vi "Read Stage Model And Serial Number.vi"(4 "error in (no error)":errorcluster, 7 "VISA resource name":refnum<visa-resource-name>) -> (0 "error out":errorcluster, 1 "Serial number":string, 2 "Model number":string, 3 "VISA resource name out":refnum<visa-resource-name>)   [LabVIEW 2020, in "Newport ESP301.lvlib"]
doc: "Reads the stage model and the serial number."
uses:
  Newport ESP301.lvlib
panel:
  in  "Axis (1)":i32=1 min=1 max=3
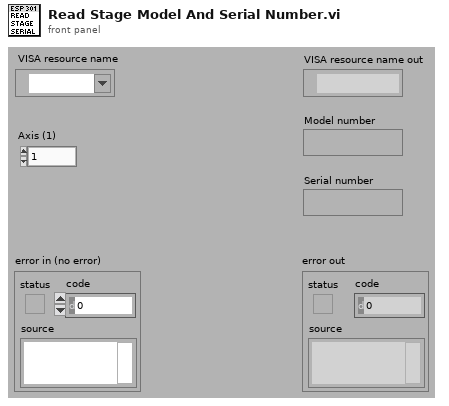
[diagram p1: front panel]
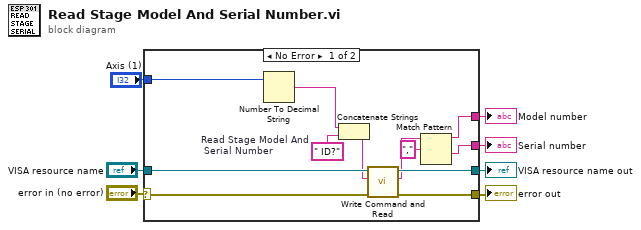
[diagram p0: block diagram]
diagram:
  n1 = case shown="No Error" "error in (no error)" {
    selector: "error in (no error)" -> [w16 w21]
    tunnel: [w18 w21] -> w7
    tunnel: "VISA resource name" -> [w19 w20]
    tunnel: [w17 w20] -> w6
    tunnel: [w12 _] -> w3
    tunnel: [w14 _] -> w2
    tunnel: "Axis (1)" -> [w10 _]
    frame No Error {
      w9 = " ID?"  # Read Stage Model And  Serial Number
      n2 = Number To Decimal String(number=w10) -> (decimal integer string=w11:string)  [unwired: 1 in]
      n3 = Concatenate Strings(w11, w9) -> (w8:string)
      n4 = call "Write Command and Read.vi"("error in (no error)"=w16, "Command"=w8, "VISA resource name"=w19) -> ("error out"=w18:errorcluster, "Returned string"=w15:string, "VISA resource name out"=w17:refnum<visa-resource-name>)  [unwired: 2 in, 2 out]
      n5 = Match Pattern(string=w15, regular expression="," ("expression régulière")) -> (before substring=w14:string, after substring=w12:string)  [unwired: 1 in, 2 out]
    }
    frame Error {
    }
  }
  "error out" <- w7
  "VISA resource name out" <- w6
  "Serial number" <- w3
  "Model number" <- w2
